vi "Response.vi"(0 "input String":string, 1 "OK":bool) -> (2 "RESPONSE":string, 3 "OK 2":bool)   [LabVIEW 2020]
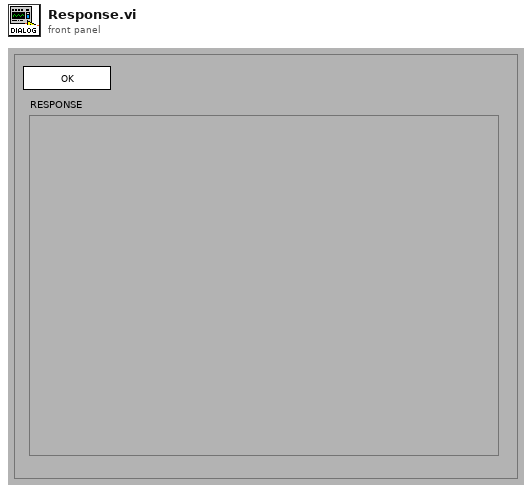
[diagram p1: front panel]
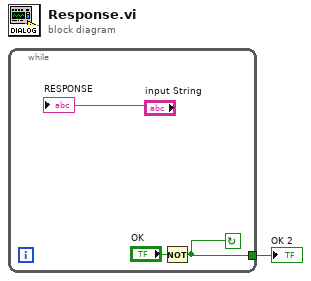
[diagram p0: block diagram]
diagram:
  n1 = while {
    tunnel: [w3] -> w1
    stop <- w3 continue-if-true
    n2 = Not(x="OK") -> (.not. x?=w3:bool)
    "RESPONSE" <- "input String"
  }
  "OK 2" <- w1
